vi "FTW-File-ListDirectory-RegexFilter.vi"(0 "Directory to Search":path, 5 "Filename Regex Filter":string="\\.vi\\z", 7 "Treat LLBs as Folders?":bool, 11 "error in":errorcluster) -> (4 "Matching Filepaths":path[](array[path]), 6 "Regex Results":cluster{"Match":string, "Submatches":string[]}[](array[cluster]), 8 "Num Files Found":i32, 15 "error out":errorcluster)   [LabVIEW 2015]
panel:
  # "Inputs"
  # "Outputs"
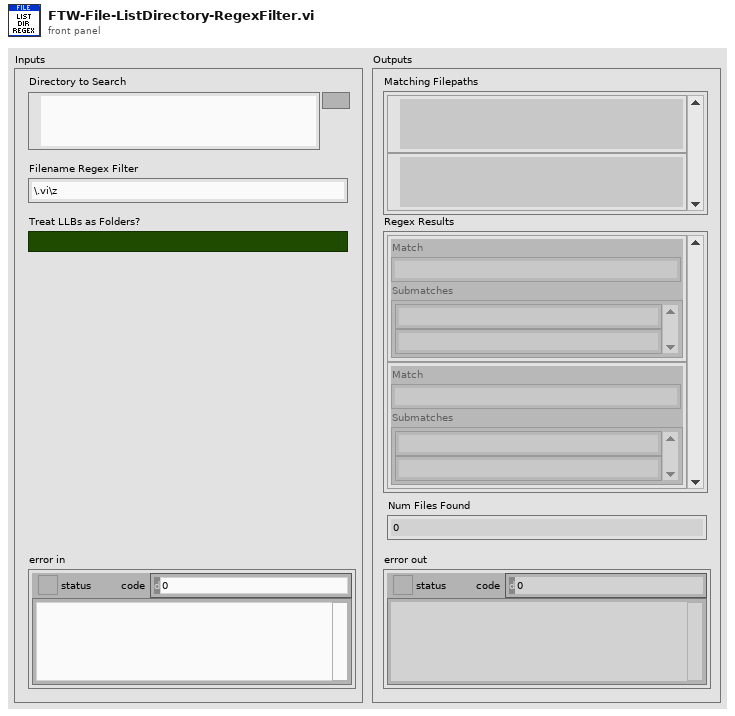
[diagram p1: front panel]
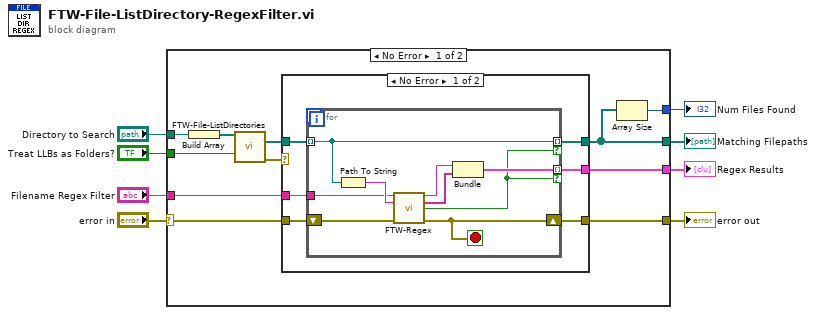
[diagram p0: block diagram]
diagram:
  n1 = case shown="No Error" "error in" {
    selector: "error in" -> [w17 w36]
    tunnel: "Filename Regex Filter" -> [w19 _]
    tunnel: "Directory to Search" -> [w18 _]
    tunnel: [w16 w36] -> w7
    tunnel: [w10 _] -> w6
    tunnel: [w11 _] -> w3
    tunnel: "Treat LLBs as Folders?" -> [w15 _]
    tunnel: [w9 _] -> w1
    frame No Error {
      n2 = Build Array(w18) -> (w12:path[])
      n3 = call "FTW-File-ListDirectories.vi"("Directories"=w12, "Treat LLBs as Folders?"=w15) -> ("Matching Filepaths"=w14:path[], "error out"=w13:errorcluster)  [unwired: 11 in, 1 out]
      n4 = case shown="No Error" w13 {
        tunnel: [w25 _] -> w11
        tunnel: w14 -> [w21 _]
        tunnel: w19 -> [w24 _]
        tunnel: w17 -> [w23 w35]
        tunnel: [w22 w35] -> w16
        tunnel: [w20 _] -> w10
        frame No Error {
          n5 = for {
            tunnel: w21 -> [w27] mode=indexing
            tunnel: [w34] -> w25 mode=indexing if=w26
            tunnel: w24 -> [w31]
            shift-right: [w30] -> w22
            shift-left: w23 -> [w32]
            tunnel: [w27] -> w20 mode=indexing if=w26
            stop <- w30 stop-if-true
            n6 = Path To String(path=w27) -> (string=w33:string)
            n7 = call "FTW-Regex.vi"("Regular Expression"=w31, "Input String"=w33, "error in"=w32) -> ("Match"=w29:string, "Submatches"=w28:string[], "Match Found?"=w26:bool, "error out"=w30:errorcluster)  [unwired: 8 in, 1 out]
            n8 = Bundle("Match"=w29, "Submatches"=w28) -> (w34:cluster{"Match":string, "Submatches":string[]})  [unwired: 1 in]
          }
        }
        frame Error {
          # "If it's an error.... we don't really\ncare. It's likely that the directory\ndid not exist."
        }
      }
      n9 = Array Size(array=w10) -> (size(s)=w9:i32)
    }
    frame Error {
    }
  }
  "error out" <- w7
  "Matching Filepaths" <- w6
  "Regex Results" <- w3
  "Num Files Found" <- w1
